vi "PanelFactory.vi"(8 "error in (no error)":errorcluster, 10 "ThreadName(\"\")":string, 11 "Member_Actor in":refnum<class "Member_Actor.lvclass">) -> (0 "error out":errorcluster, 2 "MemberPanel(Product)":refnum<class "MemberPanel.lvclass">, 3 "Member_Actor out":refnum<class "Member_Actor.lvclass">)   [LabVIEW 2015, in "Member_Actor.lvlib" / "Member_Actor.lvclass"]
uses:
  Member_Actor.lvclass
  MemberPanel/MemberPanel.lvclass
  ExcuseNote/ExcuseNote.lvclass
  Member_Actor.lvclass/Member_Actor.ctl
  ExcuseNote/ExcuseNote.lvclass/ExcuseNote.ctl
  MemberInfo/Information.lvclass
  MemberInfo/Information.lvclass/Information.ctl
  MemberTable/TimeTable.lvclass
  MemberTable/TimeTable.lvclass/TimeTable.ctl
  <vilib>/Utility/error.llb/Error Cluster From Error Code.vi
  <vilib>/ErrorRing/Error Ring.xnode
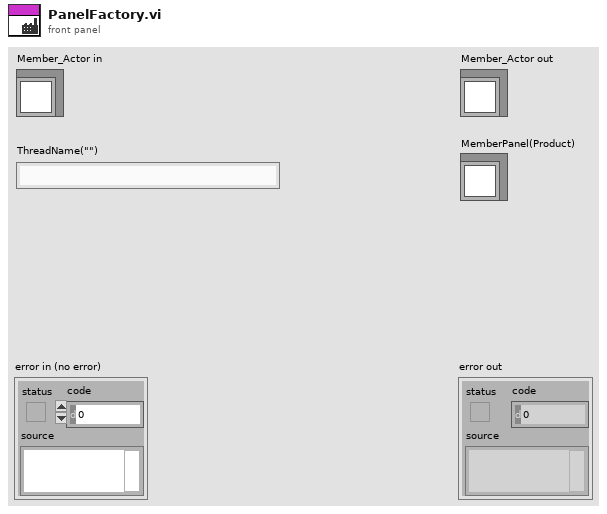
[diagram p1: front panel]
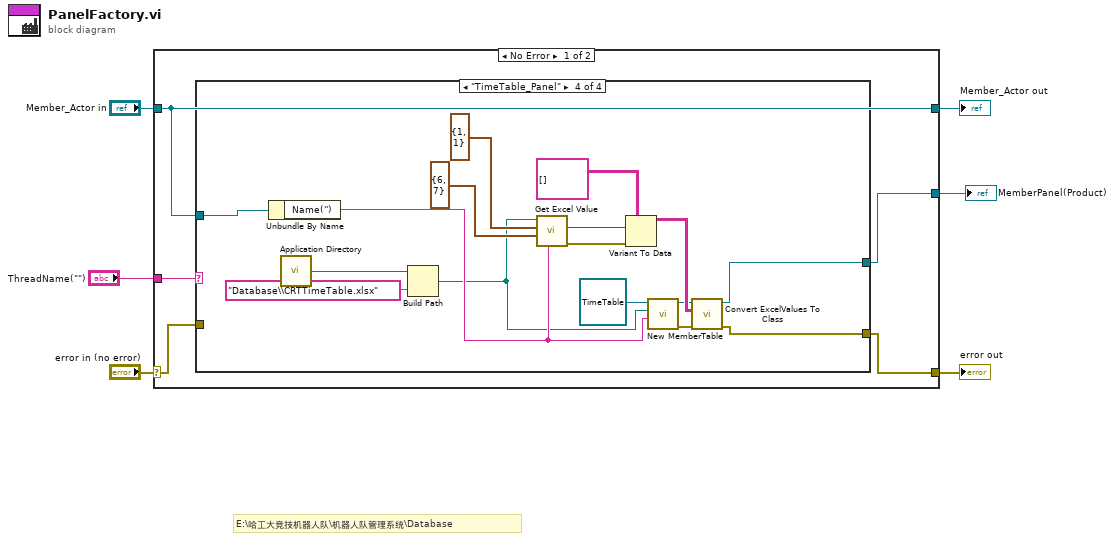
[diagram p0: block diagram]
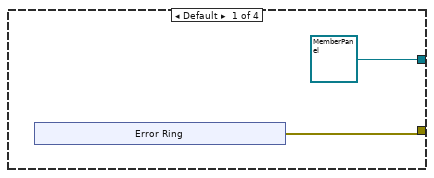
[diagram p2: hidden frame]
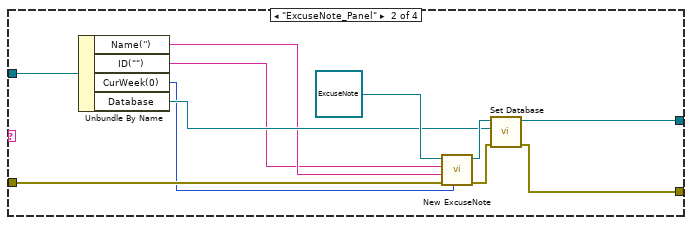
[diagram p3: hidden frame]
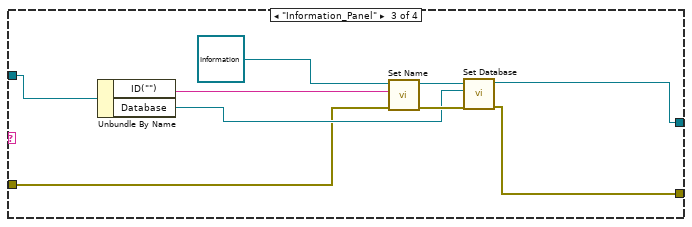
[diagram p4: hidden frame]
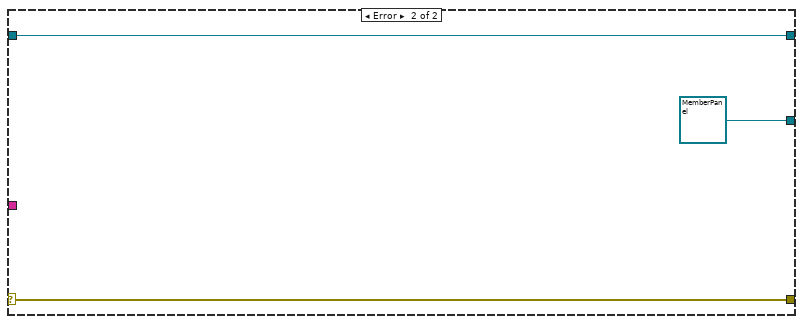
[diagram p5: hidden frame]
diagram:
  # "E:\\哈工大竞技机器人队\\机器人队管理系统\\Database"
  n1 = case shown="No Error" "error in (no error)" {
    selector: "error in (no error)" -> [w10 w57]
    tunnel: [w9 w57] -> w5
    tunnel: [w8 w56] -> w3
    tunnel: "Member_Actor in" -> [w8 w56]
    tunnel: "ThreadName(\"\")" -> [w11 _]
    tunnel: [w7 refnum<class "MemberPanel.lvclass"> refnum ("MemberInfo out")] -> w1
    frame No Error {
      n2 = case shown="\"TimeTable_Panel\"" w11 {
        tunnel: w10 -> [_ w25 w32 _]
        tunnel: [w12 w26 w31 w40] -> w9
        tunnel: w8 -> [_ w24 w35 w45]
        tunnel: [refnum<class "MemberPanel.lvclass"> refnum ("MemberInfo out") w20 w30 w41] -> w7
        frame Default {
          n3 = xnode "Error Ring"() -> ("error out"=w12:errorcluster)
        }
        frame "ExcuseNote_Panel" {
          n4 = Unbundle By Name(w24) -> ("Name('')"=w22:string, "ID(\"\")"=w21:string, "CurWeek(0)"=w19:i32, "Database"=w23:refnum<class "Database.lvclass">)
          n5 = call "New ExcuseNote.vi"("CurWeek(0)"=w19, "error in (no error)"=w25, "Name(\"\")"=w22, "ID(\"\")"=w21, "ExcuseNote in"=refnum<class "ExcuseNote.lvclass"> refnum ("Member_Actor.lvlib:ExcuseNote.lvclass")) -> ("error out"=w29:errorcluster, "ExcuseNote out"=w28:refnum<class "ExcuseNote.lvclass">)  [unwired: 5 in]
          n6 = call "Set Database.vi"("error in (no error)"=w29, "Database"=w23, "ExcuseNote in"=w28) -> ("error out"=w26:errorcluster, "ExcuseNote out"=w20:refnum<class "ExcuseNote.lvclass">)  [unwired: 7 in]
        }
        frame "Information_Panel" {
          n7 = Unbundle By Name(w35) -> ("ID(\"\")"=w34:string, "Database"=w33:refnum<class "Database.lvclass">)
          n8 = call "Set Name.vi"("error in (no error)"=w32, "ID(\"\")"=w34, "MemberInfo in"=refnum<class "Information.lvclass"> refnum) -> ("error out"=w36:errorcluster, "MemberInfo out"=w37:refnum<class "Information.lvclass">)  [unwired: 7 in]
          n9 = call "Set Database .vi"("error in (no error)"=w36, "Database"=w33, "MemberInfo in"=w37) -> ("error out"=w31:errorcluster, "MemberInfo out"=w30:refnum<class "Information.lvclass">)  [unwired: 7 in]
        }
        frame "TimeTable_Panel" {
          n10 = Unbundle By Name(w45) -> ("Name('')"=w44:string)
          n11 = call <vilib>:"Application Directory.vi"() -> ("Application Directory"=w43:path)
          n12 = Build Path(base path=w43, name or relative path="Database\\CRTTimeTable.xlsx") -> (appended path=w39:path)
          n13 = call "Get Excel Value.vi"("SheetName(\"\")"=w44, "End"=cluster{"Column":i32, "Row":i32} {"Column"=6, "Row"=7}, "Start"=cluster{"Column":i32, "Row":i32} {"Column"=1, "Row"=1}, "path"=w39) -> ("error out"=w53:errorcluster, "Excel_Value"=w51:variant)  [unwired: 6 in]
          n14 = Variant To Data(error in=w53, type=string[][] [], Variant=w51) -> (data=w54:string[][])  [unwired: 1 out]
          n15 = call "New MemberTable.vi"("SheetName(\"\")"=w44, "Path"=w39, "MemberTable in"=refnum<class "TimeTable.lvclass"> refnum) -> ("error out"=w48:errorcluster, "MemberTable out"=w47:refnum<class "TimeTable.lvclass">)  [unwired: 7 in]
          n16 = call "Convert ExcelValues To Class.vi"("error in (no error)"=w48, "Excel Value(\"\")"=w54, "MemberTable in"=w47) -> ("error out"=w40:errorcluster, "MemberTable out"=w41:refnum<class "TimeTable.lvclass">)  [unwired: 7 in]
        }
      }
    }
    frame Error {
    }
  }
  "error out" <- w5
  "Member_Actor out" <- w3
  "MemberPanel(Product)" <- w1
